vi "extract_tdms_params.vi"(1 "Input String":string) -> (0 "Output Array":cluster{"key":string, "value":dbl}[](array[cluster]))   [LabVIEW 2019]
uses:
  <vilib>/JDP Science/JDP Science Common Utilities/JDP Utility.lvlib
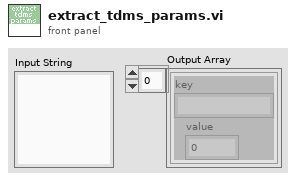
[diagram p1: front panel]
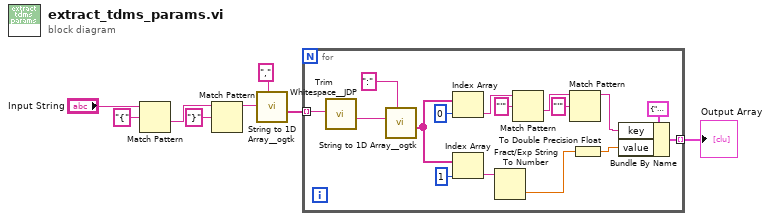
[diagram p0: block diagram]
diagram:
  n1 = Match Pattern(string="Input String", regular expression="{") -> (after substring=w5:string)  [unwired: 1 in, 3 out]
  n2 = Match Pattern(string=w5, regular expression="}") -> (before substring=w6:string)  [unwired: 1 in, 3 out]
  n3 = call <userlib>:"String to 1D Array__ogtk.vi"("delimiter (Tab)"=",", "string"=w6) -> ("Array of Strings"=w3:string[])  [unwired: 9 in]
  n4 = for {
    tunnel: w3 -> [w24] mode=indexing
    tunnel: [w17] -> w1 mode=indexing
    n5 = call <vilib>:"Trim Whitespace__JDP.vi"("String in"=w24) -> ("String out"=w23:string)  [unwired: 6 in]
    n6 = call <userlib>:"String to 1D Array__ogtk.vi"("delimiter (Tab)"=":", "string"=w23) -> ("Array of Strings"=w21:string[])  [unwired: 9 in]
    n7 = Index Array(array=w21, index=0) -> (element=w10:string)
    n8 = Index Array(array=w21, index=1) -> (element=w14:string)
    n9 = Fract/Exp String To Number(string=w14) -> (number=w15:dbl)  [unwired: 3 in, 1 out]
    n10 = Match Pattern(string=w10, regular expression="'") -> (after substring=w13:string)  [unwired: 1 in, 3 out]
    n11 = Match Pattern(string=w13, regular expression="'") -> (before substring=w9:string)  [unwired: 1 in, 3 out]
    n12 = To Double Precision Float(number=w15) -> (double precision float=w16:dbl)
    n13 = Bundle By Name(cluster=cluster{"key":string, "value":dbl} {"key"="", "value"=0.0}, "key"=w9, "value"=w16) -> (w17:cluster{"key":string, "value":dbl})
  }
  "Output Array" <- w1
